vi "SteeringMotorBlock.vi"(5 "Enum":T1(ring), 6 "STOP":bool, 7 "Speed\n (Lower than 900 counts/s)":dbl, 8 "error in (no error)":errorcluster, 9 "(Antihorario) Sentido (Horario)":bool, 10 "P":dbl, 11 "Value":dbl) -> (0 "error out":errorcluster, 3 "Waveform \nChart":dbl[][](graph))   [LabVIEW 2017]
uses:
  <vilib>/myRIO/Common/Instrument Driver Framework/myRIO v1.0/Encoder/typedefs/Encoder Signal Mode.ctl
  <vilib>/myRIO/Instrument Drivers/Onboard IO/Encoder/typedefs/Encoder Reference.ctl
  <vilib>/myRIO/Common/Instrument Driver Framework/Utilities/typedefs/myRIO Generic Hardware Reference.ctl
  <vilib>/myRIO/Common/Instrument Driver Framework/Utilities/typedefs/Hardware Version Enum.ctl
  <vilib>/myRIO/Common/Instrument Driver Framework/Utilities/typedefs/myRIO v1.0 Reference.ctl
  <vilib>/myRIO/Common/Instrument Driver Framework/Utilities/typedefs/Generic FPGA Reference.ctl
  <vilib>/myRIO/Common/Instrument Driver Framework/myRIO v1.0/Encoder/typedefs/Encoder Channels Enum.ctl
  <vilib>/myRIO/Common/Instrument Driver Framework/myRIO v1.0/Encoder/typedefs/Encoder Configuration v1.0.ctl
  <vilib>/userdefined/High Color/nirio_resource_hc.ctl
  <vilib>/myRIO/Instrument Drivers/Onboard IO/DIO/typedefs/DIO Reference.ctl
  <vilib>/myRIO/Common/Instrument Driver Framework/myRIO v1.0/DIO/typedefs/DIO Channels List.ctl
  <vilib>/myRIO/Common/Instrument Driver Framework/myRIO v1.0/DIO/typedefs/DIO Channels Enum.ctl
  <vilib>/myRIO/Instrument Drivers/Onboard IO/PWM/typedefs/PWM Reference.ctl
  <vilib>/myRIO/Common/Instrument Driver Framework/myRIO v1.0/PWM/typedefs/PWM Channels Enum.ctl
  <vilib>/myRIO/Instrument Drivers/Onboard IO/PWM/typedefs/PWM Configuration.ctl
  <vilib>/myRIO/Common/Instrument Driver Framework/Utilities/vis/Is FPGA Ref Available.vi
  <vilib>/myRIO/Common/Instrument Driver Framework/myRIO v1.0/Encoder/vis/myRIO v1.1 Open Encoder.vi
  <vilib>/myRIO/Instrument Drivers/Onboard IO/Encoder/vis/Read.vi
  <vilib>/myRIO/Common/Instrument Driver Framework/myRIO v1.0/DIO/vis/myRIO v1.1 Open DIO.vi
  <vilib>/myRIO/Instrument Drivers/Onboard IO/DIO/vis/Write.vi
  <vilib>/myRIO/Common/Instrument Driver Framework/myRIO v1.0/PWM/vis/myRIO v1.1 Open PWM.vi
  <vilib>/myRIO/Instrument Drivers/Onboard IO/PWM/vis/Set Duty Cycle and Frequency.vi
  <vilib>/myRIO/Common/Instrument Driver Framework/Utilities/vis/Validate Channels.vi
  <vilib>/myRIO/Common/Instrument Driver Framework/myRIO v1.0/Encoder/vis/myRIO v1.0 Reserve Encoder.vi
  <vilib>/myRIO/Common/Instrument Driver Framework/myRIO v1.0/DIO/vis/myRIO v1.0 Reserve DIO.vi
  <vilib>/myRIO/Common/Instrument Driver Framework/myRIO v1.0/PWM/vis/myRIO v1.0 Reserve PWM.vi
  <vilib>/myRIO/Common/Instrument Driver Framework/myRIO v1.0/Encoder/vis/myRIO v1.0 Build MUX Configuration Encoder.vi
  <vilib>/myRIO/Common/Instrument Driver Framework/myRIO v1.0/Resource Manager/vis/myRIO v1.0 Reserve Channel List.vi
  <vilib>/myRIO/Common/Instrument Driver Framework/myRIO v1.0/DIO/vis/myRIO v1.0 Build MUX Configuration DIO.vi
  <vilib>/myRIO/Common/Instrument Driver Framework/myRIO v1.0/PWM/vis/myRIO v1.0 Build MUX Configuration PWM.vi
  <vilib>/myRIO/Common/Instrument Driver Framework/myRIO v1.0/Resource Manager/vis/myRIO v1.0 Create Configuration List.vi
  <vilib>/myRIO/Common/Instrument Driver Framework/myRIO v1.0/Resource Manager/vis/myRIO v1.0 Reserve Channel.vi
  <vilib>/myRIO/Common/Instrument Driver Framework/myRIO v1.0/Resource Manager/vis/myRIO v1.0 Unreserve Channel.vi
  <vilib>/myRIO/Common/Instrument Driver Framework/myRIO v1.0/Resource Manager/vis/myRIO v1.0 Build Mutex Name.vi
  <vilib>/Utility/VariantDataType/GetNumericInfo.vi
  <vilib>/Utility/error.llb/Error Cluster From Error Code.vi
  <vilib>/myRIO/Common/Instrument Driver Framework/myRIO v1.0/myRIO v1.1 Open.vi
  <vilib>/myRIO/Common/Instrument Driver Framework/Utilities/vis/IO Manager.vi
  <vilib>/myRIO/Common/Instrument Driver Framework/Utilities/vis/Configuration Manager.vi
  <vilib>/myRIO/Common/Instrument Driver Framework/myRIO v1.0/Resource Manager/vis/myRIO v1.0 Configure IO.vi
  <vilib>/myRIO/Common/Instrument Driver Framework/myRIO v1.0/myRIO v1.0 Close.vi
  <vilib>/myRIO/Common/Instrument Driver Framework/myRIO v1.0/Encoder/vis/myRIO v1.0 Configure Encoder.vi
  <vilib>/myRIO/Common/Instrument Driver Framework/myRIO v1.0/Encoder/vis/myRIO v1.0 Read Encoder.vi
  <vilib>/myRIO/Common/Instrument Driver Framework/myRIO v1.0/DIO/vis/myRIO v1.0 Write DIO.vi
  <vilib>/myRIO/Common/Instrument Driver Framework/myRIO v1.0/PWM/vis/myRIO v1.0 Write PWM.vi
  <vilib>/myRIO/Express VI/Onboard IO/Encoder/Encoder Express VI.xnode
  <vilib>/myRIO/Instrument Drivers/Onboard IO/Encoder/vis/myRIO Encoder Open.xnode
  <vilib>/myRIO/Common/Instrument Driver Framework/myRIO v1.0/Encoder/typedefs/Encoder Count Direction Enum.ctl
  <vilib>/myRIO/Express VI/Onboard IO/DO/DO Express VI.xnode
  <vilib>/myRIO/Instrument Drivers/Onboard IO/DIO/vis/myRIO DIO Open.xnode
  <vilib>/myRIO/Express VI/Onboard IO/PWM/PWM Express VI.xnode
  <vilib>/myRIO/Instrument Drivers/Onboard IO/PWM/vis/myRIO PWM Open.xnode
  <vilib>/myRIO/Instrument Drivers/Onboard IO/Encoder/Encoder.lvlib
  <vilib>/myRIO/Instrument Drivers/Onboard IO/PWM/PWM.lvlib
  <vilib>/myRIO/Instrument Drivers/Onboard IO/DIO/DIO.lvlib
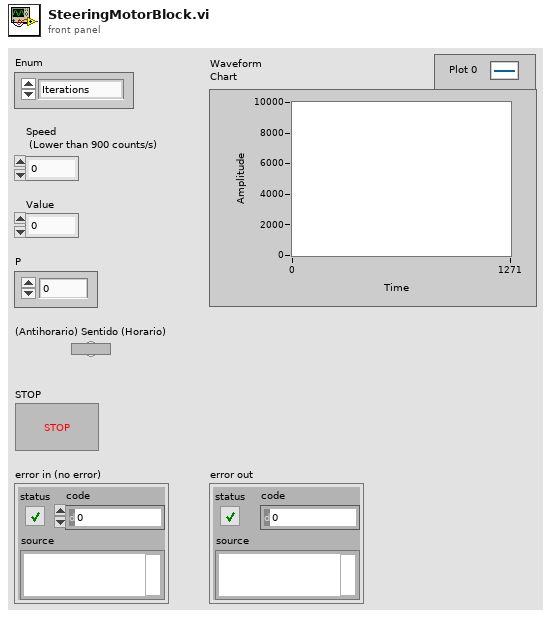
[diagram p1: front panel]
types:
  T1 = enum16{"Iterations", "Rotations", "Counts", "Degrees", "Time"}
  T2 = typedef "PWM.lvlib/PWM Reference.ctl" = cluster{"myRIO Reference":T3, "PWM Channels Enum":T7, "PWM Configuration":T8}
  T3 = typedef "myRIO Generic Hardware Reference.ctl" = cluster{"myRIO Model":T4, "myRIO Hardware Reference":T5}
  T4 = typedef "Hardware Version Enum.ctl" = enum16{"Unknown", "myRIO-1900", "myRIO-1950", "roboRIO", "NI ELVIS RIO CM"}
  T5 = typedef "myRIO v1.0 Reference.ctl" = cluster{"Generic FPGA Reference":T6, "Allow multiple opens":bool}
  T6 = typedef "Generic FPGA Reference.ctl" = refnum<k20>
  T7 = typedef "PWM Channels Enum.ctl" = enum16{"Not Connected", "C/PWM0", "C/PWM1", "A/PWM0", "A/PWM1", "A/PWM2", "B/PWM0", "B/PWM1", "B/PWM2", "PWM/PWM0", "PWM/PWM1", "PWM/PWM2", "PWM/PWM3", "PWM/PWM4", "PWM/PWM5", "PWM/PWM6", "PWM/PWM7", "PWM/PWM8", "PWM/PWM9"}
  T8 = typedef "PWM.lvlib/PWM Configuration.ctl" = cluster{"Frequency":dbl, "Duty Cycle":dbl}
  T9 = typedef "nirio_resource_hc.ctl" = tag
  T10 = typedef "Encoder.lvlib/Encoder Reference.ctl" = cluster{"myRIO Reference":T3, "Encoder Channels Enum":T11}
  T11 = typedef "Encoder Channels Enum.ctl" = enum16{"Not Connected", "C/ENC0", "C/ENC1", "A/ENC", "B/ENC", "DIO/ENC0", "DIO/ENC1", "DIO/ENC2", "DIO/ENC3", "DIO/ENC4"}
  T12 = typedef "Encoder Signal Mode.ctl" = enum16{"Quadrature phase signal", "Step and direction signal"}
  T13 = typedef "DIO.lvlib/DIO Reference.ctl" = cluster{"myRIO Reference":T3, "DIO Channels List":T14}
  T14 = typedef "DIO Channels List.ctl" = T15[]
  T15 = typedef "DIO Channels Enum.ctl" = enum16{"Not Connected", "C/DIO0", "C/DIO1", "C/DIO2", "C/DIO3", "C/DIO4", "C/DIO5", "C/DIO6", "C/DIO7", "A/DIO0", "A/DIO1", "A/DIO2", "A/DIO3", "A/DIO4", "A/DIO5", "A/DIO6", "A/DIO7", "A/DIO8", "A/DIO9", "A/DIO10", "A/DIO11", "A/DIO12", "A/DIO13", "A/DIO14", "A/DIO15", "B/DIO0", "B/DIO1", "B/DIO2", "B/DIO3", "B/DIO4", "B/DIO5", "B/DIO6", "B/DIO7", "B/DIO8", "B/DIO9", "B/DIO10", "B/DIO11", "B/DIO12", "B/DIO13", "B/DIO14", "B/DIO15", "LED0", "LED1", "LED2", "LED3", "Button0", "DIO/DIO0", "DIO/DIO1", "DIO/DIO2", "DIO/DIO3", "DIO/DIO4", "DIO/DIO5", "DIO/DIO6", "DIO/DIO7", "DIO/DIO8", "DIO/DIO9", "SPI/CS0", "SPI/CS1", "SPI/CS2", "SPI/CS3", "LED RADIO (Green)", "LED RADIO (Red)", "LED COMM (Green)", "LED COMM (Red)", "LED MODE (Green)", "LED MODE (Red)"}
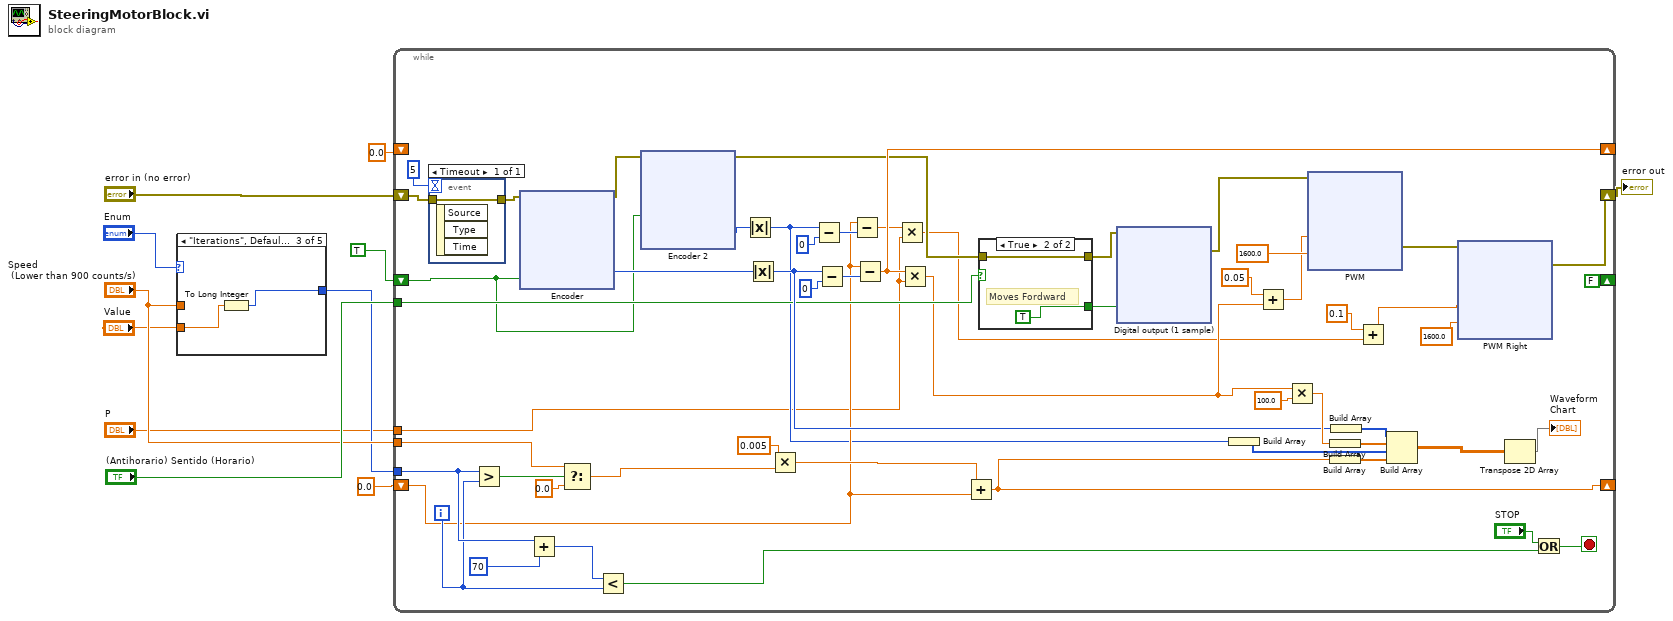
[diagram p0: block diagram]
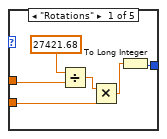
[diagram p2: hidden frame]
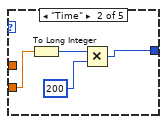
[diagram p3: hidden frame]
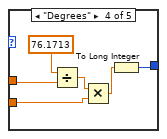
[diagram p4: hidden frame]
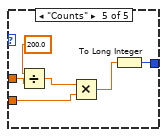
[diagram p5: hidden frame]
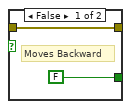
[diagram p6: hidden frame]
diagram:
  n1 = case shown="\"Iterations\", Default" "Enum" {
    tunnel: "Value" -> [w13 w18 w23 w24 w31]
    tunnel: "Speed\n (Lower than 900 counts/s)" -> [w14 _ _ w27 w34]
    tunnel: [w12 w20 w22 w29 w35] -> w9
    frame "Rotations" {
      n2 = Divide(x=27421.68 ("y"), y=w14) -> (x/y=w17:dbl)
      n3 = Multiply(x=w17, y=w13) -> (x*y=w15:dbl)
      n4 = To Long Integer(number=w15) -> (32bit integer=w12:i32)
    }
    frame "Time" {
      n5 = To Long Integer(number=w18) -> (32bit integer=w19:i32)
      n6 = Multiply(x=w19, y=200) -> (x*y=w20:i32)
    }
    frame "Iterations", Default {
      n7 = To Long Integer(number=w23) -> (32bit integer=w22:i32)
    }
    frame "Degrees" {
      n8 = Divide(x=76.1713 ("y"), y=w27) -> (x/y=w25:dbl)
      n9 = Multiply(x=w25, y=w24) -> (x*y=w28:dbl)
      n10 = To Long Integer(number=w28) -> (32bit integer=w29:i32)
    }
    frame "Counts" {
      n11 = Divide(x=200.0, y=w34) -> (x/y=w32:dbl)
      n12 = Multiply(x=w32, y=w31) -> (x*y=w30:dbl)
      n13 = To Long Integer(number=w30) -> (32bit integer=w35:i32)
    }
  }
  n14 = while {
    shift-right: [w85] -> _
    shift-left: 0.0 -> [w44]
    shift-right: [FALSE] -> _
    shift-left: TRUE -> [w52]
    tunnel: "P" -> [w36]
    shift-right: [w81] -> _
    shift-left: 0.0 -> [_]
    tunnel: "Speed\n (Lower than 900 counts/s)" -> [w82]
    shift-right: [w46] -> w5
    shift-left: "error in (no error)" -> [w68]
    tunnel: w9 -> [w63]
    tunnel: "(Antihorario) Sentido (Horario)" -> [w72]
    i -> [w60]
    stop <- w64 stop-if-true
    n15 = event shown="[0] Timeout" {
      selector: _ -> [_]
      dyn-events: _ -> [_]
      timeout: 5 -> [_]
      tunnel: [w292] -> w69
      tunnel: w68 -> [w292]
      event Timeout {
        n16 = event-data() -> ()  [unwired: 1 in, 3 out]
      }
    }
    n17 = Greater?(x=w63, y=w60) -> (0:w76:bool)
    n18 = xnode "Encoder"("Reset Counter"=w52, "error in (no error)"=w69) -> ("Counter Value"=w80:i32, "error out"=w54:errorcluster)  [unwired: 2 out]
    n19 = Add(x=w63, y=70) -> (x+y=w61:i32)
    n20 = Select(t=w82, s=w76, f=0.0) -> (s? t:f=w89:dbl)
    n21 = Less?(x=w61, y=w60) -> (x < y?=w65:bool)
    n22 = xnode "Encoder 2"("Reset Counter"=w52, "error in (no error)"=w54) -> ("Counter Value"=w48:i32, "error out"=w53:errorcluster)  [unwired: 2 out]
    n23 = Absolute Value(x=w48) -> (abs(x)=w37:i32)
    n24 = Absolute Value(x=w80) -> (abs(x)=w73:i32)
    n25 = Multiply(x=0.005 ("y"), y=w89) -> (x*y=w67:dbl)
    n26 = Subtract(x=w37, y=0) -> (x-y=w50:i32)
    n27 = Subtract(x=w73, y=0) -> (x-y=w75:i32)
    n28 = Subtract(x=w44, y=w50) -> (x-y=w49:dbl)
    n29 = Subtract(x=w44, y=w75) -> (x-y=w81:dbl)
    n30 = Multiply(x=w49, y=w36) -> (x*y=w41:dbl)
    n31 = Multiply(x=w81, y=w36) -> (x*y=w56:dbl)
    n32 = Add(x=w67, y=w44) -> (x+y=w85:dbl)
    n33 = case shown="True" w72 {
      tunnel: w53 -> [w207 w209]
      tunnel: [FALSE ("A/DIO3 (Pin 17)") TRUE ("A/DIO3 (Pin 17)")] -> w55
      tunnel: [w207 w209] -> w71
      frame False {
        # "Moves Backward"
      }
      frame True {
        # "Moves Fordward"
      }
    }
    n34 = xnode "Digital output (1 sample)"("A/DIO2 (Pin 15)"=w55, "error in (no error)"=w71) -> ("error out"=w70:errorcluster)
    n35 = Build Array(w37) -> (w38:i32[])
    n36 = Add(x=0.05, y=w56) -> (x+y=w58:dbl)
    n37 = Multiply(x=w56, y=100.0) -> (x*y=w77:dbl)
    n38 = xnode "PWM"("Duty Cycle"=w58, "Frequency [Hz]"=1600.0 ("Duty Cycle"), "error in (no error)"=w70) -> ("error out"=w47:errorcluster)
    n39 = Build Array(w77) -> (w39:dbl[])
    n40 = Build Array(w85) -> (w84:dbl[])
    n41 = Build Array(w73) -> (w40:i32[])
    n42 = Add(x=0.1, y=w41) -> (x+y=w42:dbl)
    n43 = Build Array(w40, w39, w38, w84) -> (w83:dbl[][])
    n44 = xnode "PWM Right"("Duty Cycle"=w42, "Frequency [Hz]"=1600.0, "error in (no error)"=w47) -> ("error out"=w46:errorcluster)
    n45 = Transpose 2D Array(2D array=w83) -> (transposed array=→"Waveform \nChart":dbl[][])
    n46 = Or(x="STOP", y=w65) -> (x .or. y?=w64:bool)
  }
  "error out" <- w5
